vi "DeviceInitialize.vi"(8 "error in (no error)":errorcluster, 9 "Reset (True)":bool=TRUE, 10 "ID Query (True)":bool=TRUE, 11 "TesteractHAL_DigitalOutput_NIDAQmx In":refnum<class "TesteractHAL_DigitalOutput_NIDAQmx.lvclass">) -> (0 "error out":errorcluster, 3 "TesteractHAL_DigitalOutput_NIDAQmx Out":refnum<class "TesteractHAL_DigitalOutput_NIDAQmx.lvclass">)   [LabVIEW 2017, in "TesteractHAL_DigitalOutput_NIDAQmx.lvlib" / "TesteractHAL_DigitalOutput_NIDAQmx.lvclass"]
doc: "Sets up the DAQ task as a DigitalInput or DigitalOutput. It then starts the Task.\n\nIf Reset is true the device will be reset."
uses:
  TesteractHAL_DigitalOutput_NIDAQmx.lvclass
  TesteractHAL_DigitalOutput_NIDAQmx.lvclass/TesteractHAL_DigitalOutput_NIDAQmx.ctl
  <resource>/objmgr/daqmx.rc
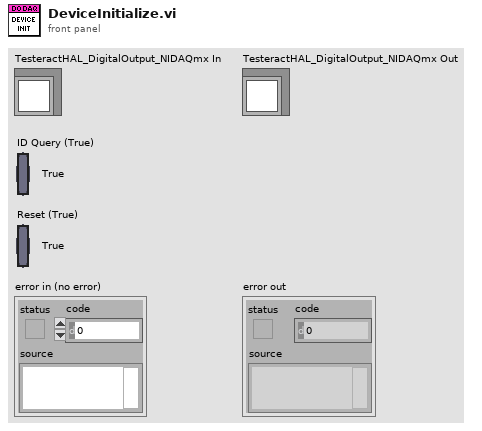
[diagram p1: front panel]
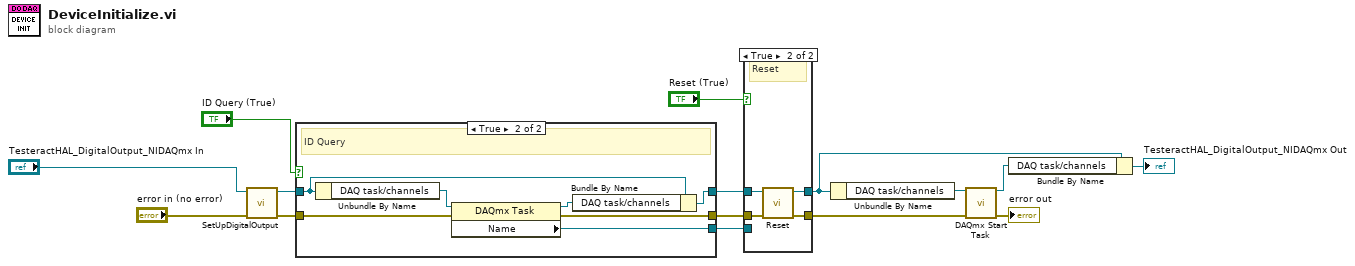
[diagram p0: block diagram]
diagram:
  n1 = call "SetUpDigitalOutput.vi"("error in (no error)"="error in (no error)", "TesteractHAL_DigitalOutput_NIDAQmx In"="TesteractHAL_DigitalOutput_NIDAQmx In") -> ("error out"=w2:errorcluster, "TesteractHAL_DigitalOutput_NIDAQmx Out"=w1:refnum<class "TesteractHAL_DigitalOutput_NIDAQmx.lvclass">)  [unwired: 8 in]
  n2 = case shown="True" "ID Query (True)" {
    tunnel: [w16 w24] -> w15
    tunnel: w2 -> [w16 w22]
    tunnel: [_ w21] -> w13
    tunnel: w1 -> [w17 w19]
    tunnel: [w17 w18] -> w12
    frame False {
      # "No ID Query"
    }
    frame True {
      # "ID Query"
      n3 = Unbundle By Name(w19) -> ("DAQ task/channels"=w23:refnum<k21>)
      n4 = property class="DAQmx Task"(reference=w23, error in=w22) -> (reference out=w20:refnum<k21>, error out=w24:errorcluster, "Name"=w21:refnum<k21>)
      n5 = Bundle By Name(cluster=w19, "DAQ task/channels"=w20) -> (w18:refnum<class "TesteractHAL_DigitalOutput_NIDAQmx.lvclass">)
    }
  }
  n6 = case shown="True" "Reset (True)" {
    tunnel: w15 -> [w26 w29]
    tunnel: [w26 w27] -> w6
    tunnel: w13 -> [_ _]
    tunnel: w12 -> [w25 w30]
    tunnel: [w25 w28] -> w8
    frame False {
      # "Don't Reset"
    }
    frame True {
      # "Reset"
      n7 = call-dynamic "Reset.vi"("error in (no error)"=w29, "TesteractHAL_DigitalOutput_NIDAQmx In"=w30) -> ("error out"=w27:errorcluster, "TesteractHAL_DigitalOutput_NIDAQmx Out"=w28:refnum<class "TesteractHAL_DigitalOutput_NIDAQmx.lvclass">)  [unwired: 8 in]
    }
  }
  n8 = Unbundle By Name(w8) -> ("DAQ task/channels"=w9:refnum<k21>)
  n9 = call <vilib>:"DAQmx Start Task.vi"("task/channels in"=w9, "error in"=w6) -> ("task out"=w7:refnum<k21>, "error out"=→"error out":errorcluster)  [unwired: 12 in]
  n10 = Bundle By Name(cluster=w8, "DAQ task/channels"=w7) -> (→"TesteractHAL_DigitalOutput_NIDAQmx Out":refnum<class "TesteractHAL_DigitalOutput_NIDAQmx.lvclass">)
